vi "Constructor.vi"(8 "error in":errorcluster, 11 "Owlstone Gen-SYS in":refnum<class "Owlstone GEN-SYS.lvclass">) -> (0 "error out":errorcluster, 2 "Init":bool, 3 "Owlstone GEN-SYS out":refnum<class "Owlstone GEN-SYS.lvclass">)   [LabVIEW 2011, in "Owlstone GEN-SYS.lvclass"]
uses:
  Owlstone GEN-SYS.lvclass
  Owlstone GEN-SYS.lvclass/Owlstone GEN-SYS.ctl
  Michell Easidew/Michell Easidew.lvclass
  Eurotherm 3200 PID Controller/Eurotherm 3200 PID Controller.lvclass
  Set Remote PID Setpoints Continuously.vi
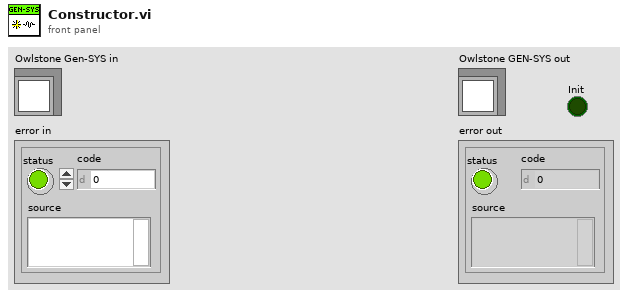
[diagram p1: front panel]
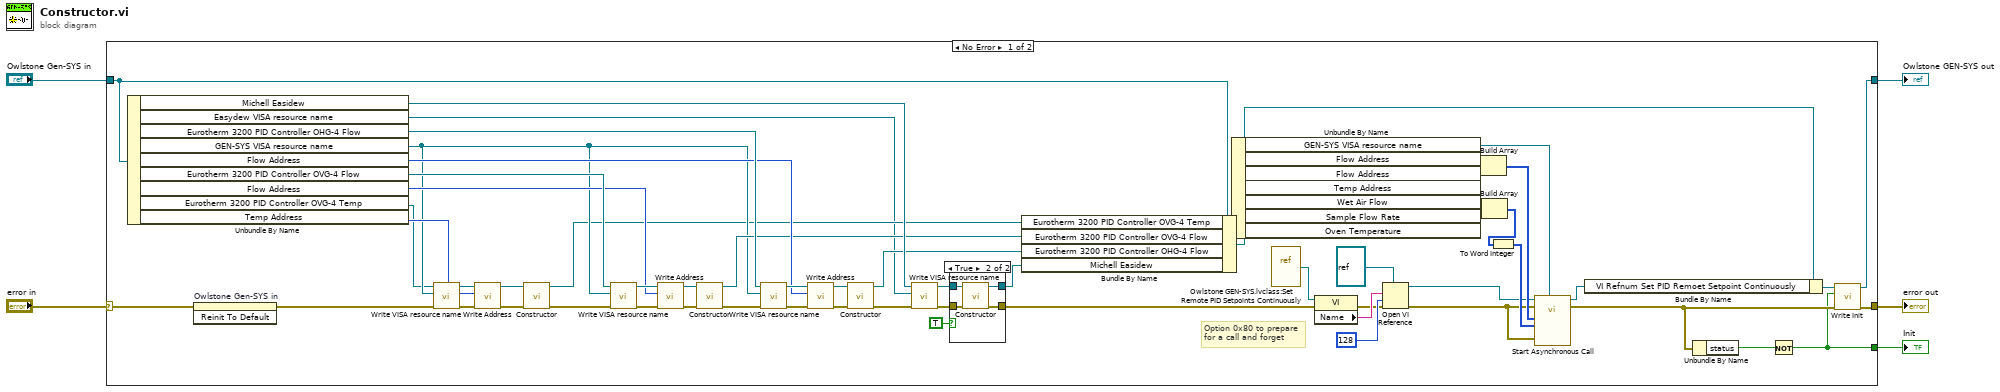
[diagram p0: block diagram]
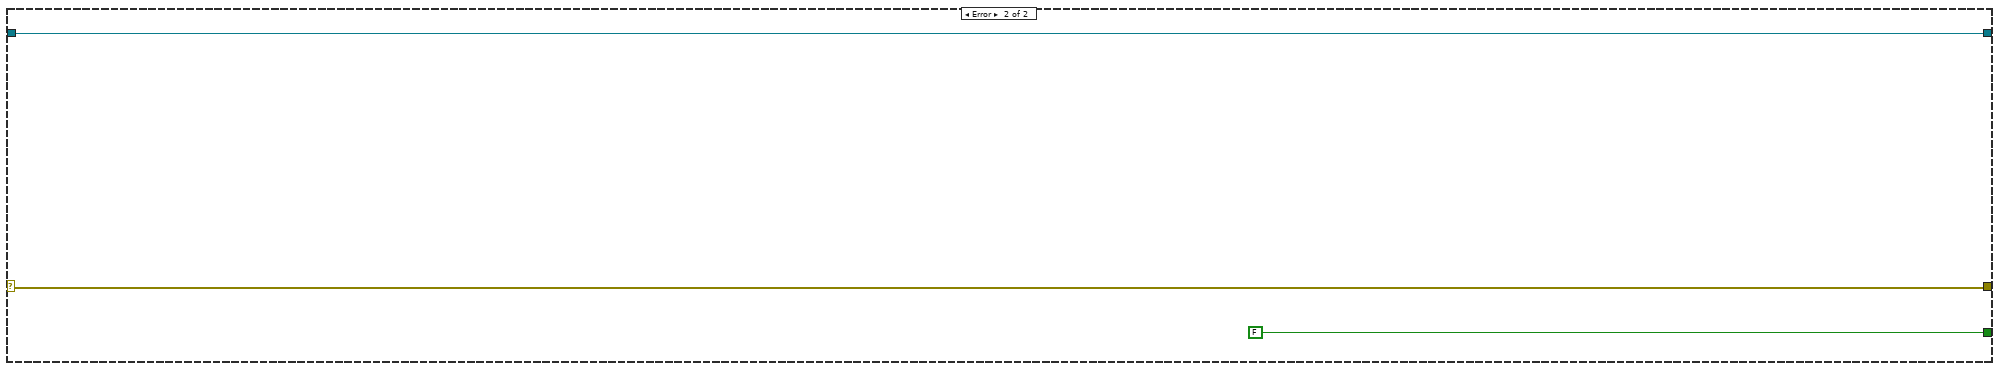
[diagram p3: hidden frame]
diagram:
  n1 = case shown="No Error" "error in" {
    selector: "error in" -> [w64 w74]
    tunnel: [w9 w74] -> w4
    tunnel: [w10 w73] -> w2
    tunnel: "Owlstone Gen-SYS in" -> [w63 w73]
    tunnel: [w8 FALSE] -> w1
    frame No Error {
      # "Option 0x80 to prepare\nfor a call and forget"
      n2 = Unbundle By Name(w63) -> ("Michell Easidew"=w62:refnum<class "Michell Easidew.lvclass">, "Easydew VISA resource name"=w27:refnum<visa-resource-name>, "Eurotherm 3200 PID Controller OHG-4 Flow"=w59:refnum<class "Eurotherm 3200 PID Controller.lvclass">, "GEN-SYS VISA resource name"=w35:refnum<visa-resource-name>, "Flow Address"=w57:u8, "Eurotherm 3200 PID Controller OVG-4 Flow"=w46:refnum<class "Eurotherm 3200 PID Controller.lvclass">, "Flow Address"=w45:u8, "Eurotherm 3200 PID Controller OVG-4 Temp"=w34:refnum<class "Eurotherm 3200 PID Controller.lvclass">, "Temp Address"=w36:u8)
      n3 = invoke on="Owlstone Gen-SYS in" class="LVClassControl (strict)" method="Reinit To Default"(error in=w64) -> (error out=w37:errorcluster)  [unwired: 2 in, 2 out]
      n4 = call-dynamic "Write VISA resource name.vi"("error in (no error)"=w37, "VISA resource name"=w35, "Eurotherm 3200 PID Controller in"=w34) -> ("error out"=w43:errorcluster, "Eurotherm 3200 PID Controller out"=w44:refnum<class "Eurotherm 3200 PID Controller.lvclass">)  [unwired: 7 in]
      n5 = call-dynamic "Write Address.vi"("error in (no error)"=w43, "Address"=w36, "Eurotherm 3200 PID Controller in"=w44) -> ("error out"=w42:errorcluster, "Eurotherm 3200 PID Controller out"=w41:refnum<class "Eurotherm 3200 PID Controller.lvclass">)  [unwired: 7 in]
      n6 = call-dynamic "Constructor.vi"("error in (no error)"=w42, "Eurotherm 3200 PID Controller in"=w41) -> ("error out"=w40:errorcluster, "Eurotherm 3200 PID Controller out"=w33:refnum<class "Eurotherm 3200 PID Controller.lvclass">)  [unwired: 8 in]
      n7 = call-dynamic "Write VISA resource name.vi"("error in (no error)"=w40, "VISA resource name"=w35, "Eurotherm 3200 PID Controller in"=w46) -> ("error out"=w50:errorcluster, "Eurotherm 3200 PID Controller out"=w51:refnum<class "Eurotherm 3200 PID Controller.lvclass">)  [unwired: 7 in]
      n8 = call-dynamic "Write Address.vi"("error in (no error)"=w50, "Address"=w45, "Eurotherm 3200 PID Controller in"=w51) -> ("error out"=w49:errorcluster, "Eurotherm 3200 PID Controller out"=w48:refnum<class "Eurotherm 3200 PID Controller.lvclass">)  [unwired: 7 in]
      n9 = call-dynamic "Constructor.vi"("error in (no error)"=w49, "Eurotherm 3200 PID Controller in"=w48) -> ("error out"=w47:errorcluster, "Eurotherm 3200 PID Controller out"=w38:refnum<class "Eurotherm 3200 PID Controller.lvclass">)  [unwired: 8 in]
      n10 = call-dynamic "Write VISA resource name.vi"("error in (no error)"=w47, "VISA resource name"=w35, "Eurotherm 3200 PID Controller in"=w59) -> ("error out"=w56:errorcluster, "Eurotherm 3200 PID Controller out"=w58:refnum<class "Eurotherm 3200 PID Controller.lvclass">)  [unwired: 7 in]
      n11 = call-dynamic "Write Address.vi"("error in (no error)"=w56, "Address"=w57, "Eurotherm 3200 PID Controller in"=w58) -> ("error out"=w55:errorcluster, "Eurotherm 3200 PID Controller out"=w54:refnum<class "Eurotherm 3200 PID Controller.lvclass">)  [unwired: 7 in]
      n12 = call-dynamic "Constructor.vi"("error in (no error)"=w55, "Eurotherm 3200 PID Controller in"=w54) -> ("error out"=w52:errorcluster, "Eurotherm 3200 PID Controller out"=w53:refnum<class "Eurotherm 3200 PID Controller.lvclass">)  [unwired: 8 in]
      n13 = call-dynamic "Write VISA resource name.vi"("error in (no error)"=w52, "VISA resource name"=w27, "Michell Easydew in"=w62) -> ("error out"=w61:errorcluster, "Michell Easydew out"=w60:refnum<class "Michell Easidew.lvclass">)  [unwired: 7 in]
      n14 = case shown="True" TRUE {
        tunnel: w61 -> [w67 w71]
        tunnel: w60 -> [w66 w70]
        tunnel: [w66 w69] -> w39
        tunnel: [w67 w68] -> w16
        frame False {
        }
        frame True {
          n15 = call-dynamic "Constructor.vi"("error in (no error)"=w71, "Michell Easydew in"=w70) -> ("error out"=w68:errorcluster, "Michell Easydew out"=w69:refnum<class "Michell Easidew.lvclass">)  [unwired: 8 in]
        }
      }
      n16 = Bundle By Name(cluster=w63, "Eurotherm 3200 PID Controller OVG-4 Temp"=w33, "Eurotherm 3200 PID Controller OVG-4 Flow"=w38, "Eurotherm 3200 PID Controller OHG-4 Flow"=w53, "Michell Easidew"=w39) -> (w18:refnum<class "Owlstone GEN-SYS.lvclass">)
      n17 = Unbundle By Name(w18) -> ("GEN-SYS VISA resource name"=w19:refnum<visa-resource-name>, "Flow Address"=w23:u8, "Flow Address"=w22:u8, "Temp Address"=w21:u8, "Wet Air Flow"=w24:i32, "Sample Flow Rate"=w25:i32, "Oven Temperature"=w26:i32)
      n18 = vi-ref "Owlstone GEN-SYS.lvclass:Set Remote PID Setpoints Continuously.vi"() -> (w31:refnum<vi>)
      n19 = property class="VI"(reference=w31, error in=w16) -> (error out=w29:errorcluster, "Name"=w32:string)  [unwired: 1 out]
      n20 = Open VI Reference(type specifier VI Refnum (for type only)=refnum<vi> refnum, vi path=w32, options=128, error in (no error)=w29) -> (vi reference=w7:refnum<vi>, error out=w6:errorcluster)  [unwired: 2 in]
      n21 = Build Array(w23, w22, w21) -> (w20:u8[])
      n22 = Build Array(w24, w25, w26) -> (w15:i32[])
      n23 = To Word Integer(number=w15) -> (16bit integer=w14:i16[])
      n24 = call-by-ref "Start Asynchronous Call"(reference=w7, error in=w6, "VISA resource name"=w19, "error in"=w6, "Remote Setpoint"=w14, "Unit Addresses"=w20) -> (reference out=w17:refnum<vi>, error out=w12:errorcluster)  [unwired: 7 in, 1 out]
      n25 = Bundle By Name(cluster=w18, "VI Refnum Set PID Remoet Setpoint Continuously"=w17) -> (w11:refnum<class "Owlstone GEN-SYS.lvclass">)
      n26 = Unbundle By Name(w12) -> ("status"=w65:bool)
      n27 = Not(x=w65) -> (.not. x?=w8:bool)
      n28 = call-dynamic "Write Init.vi"("error in (no error)"=w12, "Init"=w8, "Vapour Generator in"=w11) -> ("error out"=w9:errorcluster, "Vapour Generator out"=w10:refnum<class "Owlstone GEN-SYS.lvclass">)  [unwired: 7 in]
    }
    frame Error {
    }
  }
  "error out" <- w4
  "Owlstone GEN-SYS out" <- w2
  "Init" <- w1
